vi "Open IPS.vi"(8 "error in (no error)":errorcluster, 11 "Instrument.Oxford1820 in":refnum<class "Instrument.Oxford1820.lvclass">) -> (0 "error out":errorcluster, 3 "Instrument.Oxford1820 out":refnum<class "Instrument.Oxford1820.lvclass">)   [LabVIEW 2016, in "Instrument.Oxford1820.lvclass"]
uses:
  Instrument.Oxford1820.lvclass
  <instrlib>/Mercury iXX/Public/Controls/Comms Transport Layer.ctl
  Instrument.Oxford1820.lvclass/Instrument.Oxford1820.ctl
  <instrlib>/Mercury iXX/Public/Libraries/System/Open/Open System.vi
  <instrlib>/Mercury iXX/Public/Libraries/System/Read/Catalogue (Read).vi
  <instrlib>/Mercury iXX/Mercury iXX.lvlib
  <instrlib>/Mercury iXX/Public/Libraries/System.lvlib
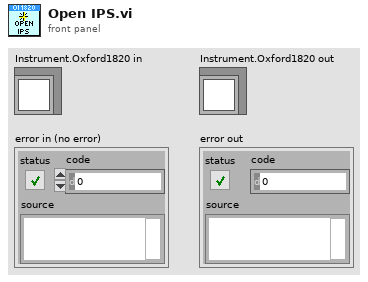
[diagram p1: front panel]
types:
  T1 = typedef "Mercury iXX.lvlib/Comms Transport Layer.ctl" = enum16{"Ethernet TCP/IP", "USB", "ISOBus - RS-232", "GPIB"}
  T2 = typedef "Mercury iXX.lvlib/Mercury Reference.ctl" = cluster{"Comms":refnum<visa-resource-name>, "Device ID":string[], "Comms Layer":T1, "Command":string, "Query reference":T3}
  T3 = typedef "Mercury iXX.lvlib/Query Dynamic Reference.ctl" = refnum<vi>
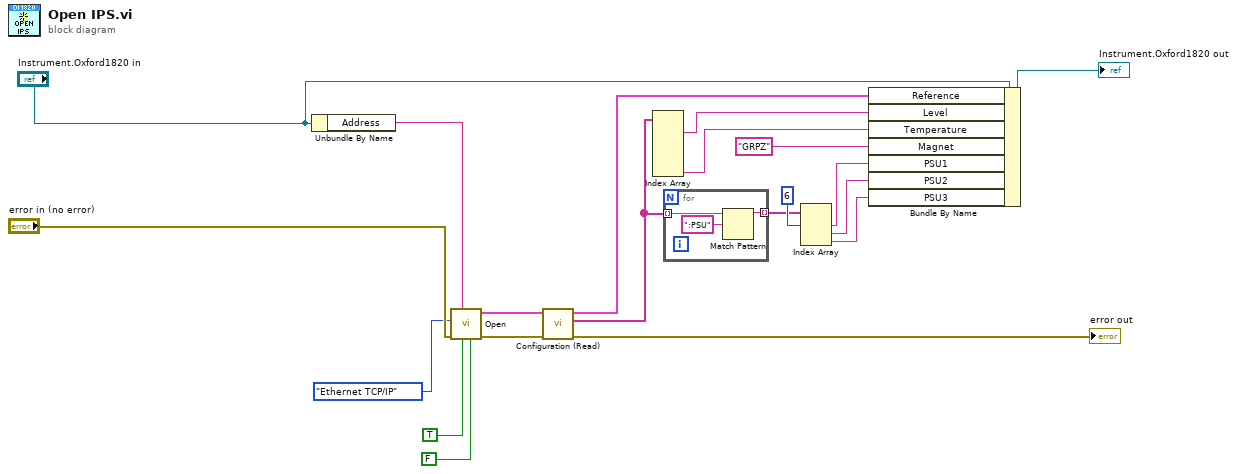
[diagram p0: block diagram]
diagram:
  n1 = Unbundle By Name("Instrument.Oxford1820 in") -> ("Address"=w4:string)
  n2 = call-poly <instrlib>:"Open.vi"("Clear Previous Connections (False)"=FALSE, "ID Query (True)"=TRUE, "IP Address"=w4, "error in (no error)"="error in (no error)", "Comms Layer"=Comms_Transport_Layer."Ethernet TCP/IP") -> ("error out"=w6:errorcluster, "Mercury Reference Out"=w7:T2)  [unwired: 2 in, 3 out]
  n3 = call-poly <instrlib>:"Configuration (Read).vi"("error in"=w6, "Mercury Reference In"=w7) -> ("error out"=→"error out":errorcluster, "Devices"=w14:string[], "Mercury Reference Out"=w9:T2)  [unwired: 1 in, 6 out]
  n4 = Index Array(array=w14) -> (element #1=w11:string, element #6=w1:string)  [unwired: 6 in, 4 out]
  n5 = for {
    tunnel: w14 -> [w22] mode=indexing
    tunnel: [w21] -> w12 mode=indexing
    n6 = Match Pattern(string=w22, regular expression=":PSU") -> (before substring=w21:string)  [unwired: 1 in, 3 out]
  }
  n7 = Index Array(array=w12, index #1=6 ("index")) -> (element #1=w16:string, element #2=w17:string, element #3=w18:string)  [unwired: 2 in]
  n8 = Bundle By Name(cluster="Instrument.Oxford1820 in", "Reference"=w9, "Level"=w11, "Temperature"=w1, "Magnet"="GRPZ" ("IPS.Devices.Magnet (GRPZ)"), "PSU1"=w16, "PSU2"=w17, "PSU3"=w18) -> (→"Instrument.Oxford1820 out":refnum<class "Instrument.Oxford1820.lvclass">)
